vi "HOST_timecycleAIstreaming_11-9.vi"() -> ()   [LabVIEW 2020]
uses:
  <vilib>/rvi/interface/nirviMethod/nirviMethod.xnode
  <vilib>/rvi/errors/niLvFpgaMergeErrorWithErrorCode.vi
  <instrlib>/_niInstr/Streaming/v1/Host/niInstr Streaming v1 Host.lvlib
  <vilib>/rvi/interface/nirviReadWriteControl/nirviReadWriteControl.xnode
  <vilib>/rvi/interface/nirviCloseFPGA/nirviCloseFPGA.xnode
  <vilib>/rvi/interface/nirviOpenFPGA/nirviOpenFPGA.xnode
  <vilib>/rvi/interface/Simulation/niFpgaSimulationCallBeginRW.vi
  <vilib>/rvi/errors/niLvFpgaAdjustHostInterfaceError.vi
  <instrlib>/_niInstr/Streaming/v1/Host/Public/Start Continuous Stream.vi
  <instrlib>/_niInstr/Streaming/v1/Host/Public/Wait for Stream.vi
  <instrlib>/_niInstr/Streaming/v1/Host/Public/Start Finite Stream.vi
  <vilib>/rvi/Analysis/host/Butterworth/config/Butterworth Filter Order.ctl
  <vilib>/rvi/Analysis/host/Public/NI_FpgaMspHost.lvlib
  <vilib>/rvi/Analysis/host/Butterworth/config/Butterworth Filter Type.ctl
  <vilib>/rvi/Analysis/host/Butterworth/config/BwScaledCoefficients.vi
  <vilib>/rvi/Analysis/host/Butterworth/XNode/ButterworthCoefficients.xnode
  FPGA Bitfiles/rfsignal_FPGATarget_TimecyclingNoMod_q9dttbL5ptg.lvbitx
  <vilib>/FPGAPlugInAG/PXIe-7972R/niLvFpga_Open_PXIe-7972R.vi
  <vilib>/rvi/interface/common/dynamic/niFpgaDynamicAddResources.vi
  <vilib>/FPGAPlugInAG/Dynamic/niLvFpga_ConfigureFifo_Dynamic.vi
  <vilib>/FPGAPlugInAG/Dynamic/niLvFpga_StartFifo_Dynamic.vi
  <vilib>/FPGAPlugInAG/Dynamic/niLvFpga_WriteFifo_Dynamic.vi
  <vilib>/FPGAPlugInAG/Dynamic/niLvFpga_ReadFifo_Dynamic.vi
  <vilib>/FPGAPlugInAG/Dynamic/niLvFpga_Close_Dynamic.vi
  <vilib>/userDefined/Silver/nirio_resource_slv.ctl
  Controls/Clock Select.ctl
panel:
  in  "Data Trigger Level (V)":dbl
  in  "Record Size":u16=1024
  out "AI":waveform(dbl)[](graph)
  in  "Data Trigger When":enum8{"Trigger Above", "Trigger Below"}(ring)
  in  "Trigger Type":enum8{"Immediate", "Data Trigger", "TRIG input"}(ring)
  in  "CH0 Amp inc/dec":u8[](array[ring])=[0, 0, 0, 0, 0, 0, 0, 0, 0, 0] items=["", "Increase", "Decrease"]
  in  "CH0 Freq inc/dec":u8[](array[ring])=[0, 0, 0, 0, 0, 0, 0, 0, 0, 0] items=["", "Increase", "Decrease"]
  in  "CH1 Amp inc/dec":u8[](array[ring])=[0, 0, 0, 0, 0, 0, 0, 0, 0, 0] items=["", "Increase", "Decrease"]
  in  "CH1 Freq inc/dec":u8[](array[ring])=[0, 0, 0, 0, 0, 0, 0, 0, 0, 0] items=["", "Increase", "Decrease"]
  in  "LP FF":dbl=5000.0 format="%#_13g"
  in  "Refresh Integral":bool
  in  "Setpoint Z 4":i16
  in  "Lower lim Z 4":fxp<+/-,16,16>=-300.0
  in  "Upper lim Z 4":fxp<+/-,16,16>=300.0
  in  "hp freq Z 4":dbl=1300.0
  in  "lp freq Z 4":dbl=1300.0
  in  "Setpoint Y 4":i16
  in  "Lower lim Y 4":fxp<+/-,16,16>=-300.0
  in  "Upper lim Y 4":fxp<+/-,16,16>=300.0
  in  "hp freq Y 4":dbl=1300.0
  in  "lp freq Y 4":dbl=1300.0
  in  "Setpoint X 4":i16
  in  "Lower lim X 4":fxp<+/-,16,16>=-300.0
  in  "Upper lim X 4":fxp<+/-,16,16>=300.0
  in  "hp freq X 4":dbl=1300.0
  in  "lp freq X 4":dbl=1300.0
  in  "Scaling (Z) 4":fxp<+,16,4>=1.0
  in  "Scaling (Y) 4":fxp<+,16,4>=1.0
  in  "Scaling (X) 4":fxp<+,16,4>=1.0
  in  "D (Z) 4":fxp<+/-,16,16>
  in  "I (Z) 4":fxp<+/-,16,16>
  in  "P (Z) 4":fxp<+/-,16,16>
  in  "D (Y) 4":fxp<+/-,16,16>
  in  "I (Y) 4":fxp<+/-,16,16>
  in  "P (Y) 4":fxp<+/-,16,16>
  in  "D (X) 4":fxp<+/-,16,16>
  in  "I (X) 4":fxp<+/-,16,16>
  in  "P (X) 4":fxp<+/-,16,16>
  in  "Setpoint Z 3":i16
  in  "Lower lim Z 3":fxp<+/-,16,16>=-300.0
  in  "Upper lim Z 3":fxp<+/-,16,16>=300.0
  in  "hp freq Z 3":dbl=1300.0
  in  "lp freq Z 3":dbl=1300.0
  in  "Setpoint Y 3":i16
  in  "Lower lim Y 3":fxp<+/-,16,16>=-300.0
  in  "Upper lim Y 3":fxp<+/-,16,16>=300.0
  in  "hp freq Y 3":dbl=1300.0
  in  "lp freq Y 3":dbl=1300.0
  in  "Setpoint X 3":i16
  in  "Lower lim X 3":fxp<+/-,16,16>=-300.0
  in  "Upper lim X 3":fxp<+/-,16,16>=300.0
  in  "hp freq X 3":dbl=1300.0
  in  "lp freq X 3":dbl=1300.0
  in  "Scaling (Z) 3":fxp<+,16,4>=1.0
  in  "Scaling (Y) 3":fxp<+,16,4>=1.0
  in  "Scaling (X) 3":fxp<+,16,4>=1.0
  in  "D (Z) 3":fxp<+/-,16,16>
  in  "I (Z) 3":fxp<+/-,16,16>
  in  "P (Z) 3":fxp<+/-,16,16>
  in  "D (Y) 3":fxp<+/-,16,16>
  in  "I (Y) 3":fxp<+/-,16,16>
  in  "P (Y) 3":fxp<+/-,16,16>
  in  "D (X) 3":fxp<+/-,16,16>
  in  "I (X) 3":fxp<+/-,16,16>
  in  "P (X) 3":fxp<+/-,16,16>
  in  "Setpoint Z 2":i16
  in  "Lower lim Z 2":fxp<+/-,16,16>=-300.0
  in  "Upper lim Z 2":fxp<+/-,16,16>=300.0
  in  "hp freq Z 2":dbl=1300.0
  in  "lp freq Z 2":dbl=1300.0
  in  "Setpoint Y 2":i16
  in  "Lower lim Y 2":fxp<+/-,16,16>=-300.0
  in  "Upper lim Y 2":fxp<+/-,16,16>=300.0
  in  "hp freq Y 2":dbl=1300.0
  in  "lp freq Y 2":dbl=1300.0
  in  "Setpoint X 2":i16
  in  "Lower lim X 2":fxp<+/-,16,16>=-300.0
  in  "Upper lim X 2":fxp<+/-,16,16>=300.0
  in  "hp freq X 2":dbl=1300.0
  in  "lp freq X 2":dbl=1300.0
  in  "Scaling (Z) 2":fxp<+,16,4>=1.0
  in  "Scaling (Y) 2":fxp<+,16,4>=1.0
  in  "Scaling (X) 2":fxp<+,16,4>=1.0
  in  "D (Z) 2":fxp<+/-,16,16>
  in  "I (Z) 2":fxp<+/-,16,16>
  in  "P (Z) 2":fxp<+/-,16,16>
  in  "D (Y) 2":fxp<+/-,16,16>
  in  "I (Y) 2":fxp<+/-,16,16>
  in  "P (Y) 2":fxp<+/-,16,16>
  in  "D (X) 2":fxp<+/-,16,16>
  in  "I (X) 2":fxp<+/-,16,16>
  in  "P (X) 2":fxp<+/-,16,16>
  in  "Setpoint Z 1":i16
  in  "Lower lim Z 1":fxp<+/-,16,16>=-300.0
  in  "Upper lim Z 1":fxp<+/-,16,16>=300.0
  in  "hp freq Z 1":dbl=1300.0
  in  "lp freq Z 1":dbl=1300.0
  in  "Setpoint Y 1":i16
  in  "Lower lim Y 1":fxp<+/-,16,16>=-300.0
  in  "Upper lim Y 1":fxp<+/-,16,16>=300.0
  in  "hp freq Y 1":dbl=1300.0
  in  "lp freq Y 1":dbl=1300.0
  in  "Setpoint X 1":i16
  in  "Lower lim X 1":fxp<+/-,16,16>=-300.0
  in  "Upper lim X 1":fxp<+/-,16,16>=300.0
  in  "hp freq X 1":dbl=1300.0
  in  "lp freq X 1":dbl=1300.0
  out "AI 2 beam 1":cluster{"AI0":i16, "AI3":i16}(graph)={"AI0"=37, "AI3"=37}
  out "AI 1 beam 1":cluster{"AI0":i16, "AI3":i16}(graph)={"AI0"=-70, "AI3"=-70}
  out "AI 0 beam 1":cluster{"AI0":i16, "AI3":i16}(graph)={"AI0"=-27, "AI3"=-27}
  out "Individual feedback, Z (gain)":cluster{dbl, dbl}(graph)
  out "Individual feedback, Y":cluster{dbl, dbl}(graph)
  out "Individual feedback, X 1":cluster{dbl, dbl}(graph)
  in  "Scaling (Z) 1":fxp<+,16,4>=1.0
  in  "Scaling (Y) 1":fxp<+,16,4>=1.0
  in  "Scaling (X) 1":fxp<+,16,4>=1.0
  in  "D (Z) 1":fxp<+/-,16,16>
  in  "I (Z) 1":fxp<+/-,16,16>
  in  "P (Z) 1":fxp<+/-,16,16>
  in  "D (Y) 1":fxp<+/-,16,16>
  in  "I (Y) 1":fxp<+/-,16,16>
  in  "P (Y) 1":fxp<+/-,16,16>
  in  "D (X) 1":fxp<+/-,16,16>
  in  "I (X) 1":fxp<+/-,16,16>
  in  "P (X) 1":fxp<+/-,16,16>
  out "AI 2 beam 4":cluster{"AI0":i16, "AI3":i16}(graph)
  out "AI 1 beam 4":cluster{"AI0":i16, "AI3":i16}(graph)
  out "AI 0 beam 4":cluster{"AI0":i16, "AI3":i16}(graph)
  out "AI 2 beam 3":cluster{"AI0":i16, "AI3":i16}(graph)={"AI0"=30, "AI3"=30}
  out "AI 1 beam 3":cluster{"AI0":i16, "AI3":i16}(graph)={"AI0"=-64, "AI3"=-64}
  out "AI 0 beam 3":cluster{"AI0":i16, "AI3":i16}(graph)={"AI0"=-28, "AI3"=-28}
  out "AI 2 beam 2":cluster{"AI0":i16, "AI3":i16}(graph)={"AI0"=32, "AI3"=32}
  out "AI 1 beam 2":cluster{"AI0":i16, "AI3":i16}(graph)={"AI0"=-67, "AI3"=-67}
  out "AI 0 beam 2":cluster{"AI0":i16, "AI3":i16}(graph)={"AI0"=-30, "AI3"=-30}
  out "Individual feedback, Z (gain) 4":cluster{dbl, dbl}(graph)
  out "Individual feedback, Z (gain) 3":cluster{dbl, dbl}(graph)
  out "Individual feedback, Z (gain) 2":cluster{dbl, dbl}(graph)
  out "Individual feedback, Y 4":cluster{dbl, dbl}(graph)
  out "Individual feedback, Y 3":cluster{dbl, dbl}(graph)
  out "Individual feedback, Y 2":cluster{dbl, dbl}(graph)
  out "Individual feedback, X 4":cluster{dbl, dbl}(graph)
  out "Individual feedback, X 3":cluster{dbl, dbl}(graph)
  out "Individual feedback, X 2":cluster{dbl, dbl}(graph)
  in  "Norm % 2":dbl=1.0 format="%#_13g"
  in  "Norm %":dbl=1.0 format="%#_13g"
  in  "Amp mod on/off":bool[](array[boolean])=[FALSE, FALSE, FALSE, FALSE, FALSE, FALSE, FALSE, FALSE, FALSE]
  in  "Mod Amp (%)":fxp<+,16,1>[](array[numeric])=[0.5, 1.0, 1.0, 1.0, 0.5, 1.0, 1.0, 1.0, 1.0]
  in  "Mod Fq (Hz) 3":dbl[](array[numeric])=[0.1, 1.0, 1.0, 1.0, 0.1, 1.0, 0.0, 1.0, 1.0] format="%5p"
  in  "Gain X %/s":fxp<+/-,64,32>
  in  "Gain Y %/s":fxp<+/-,64,32>
  in  "X (CH1) Hz/s":fxp<+/-,64,32>
  in  "Y (CH0) Hz/s":fxp<+/-,64,32>
  in  "Input pass through\nmode":enum16{"Wire", "Accum", "Accum-edge"}(ring)
  in  "# of beams":i8=1
  in  "Wave Reader CH 1 (X)":fxp<+/-,64,32>[](array[numeric])=[27000000.0, 26000000.0, 28000000.0, 25000000.0, 21000000.0, 25000000.0, 30000000.0, 34000000.0, 27000000.0] format="%_17p"
  in  "Gain CH 1 (multiplicative)":fxp<+,32,4>[](array[numeric])=[1.0, 1.0, 0.9999999925494194, 1.0, 1.0, 1.0, 1.0, 1.0, 1.0]
  in  "Remove transition edges":i32=5
  in  "Time per beam in us":i32=20
  in  "stop":bool
  in  "Gain CH 0 (multiplicative)":fxp<+,32,4>[](array[numeric])=[1.0, 1.0, 1.0, 1.0, 1.0, 1.0, 1.0, 1.0, 1.0]
  in  "Wave Reader CH 0 (Y)":fxp<+/-,64,32>[](array[numeric])=[27000000.0, 26000000.0, 28000000.0, 25000000.0, 21000000.0, 25000000.0, 30000000.0, 34000000.0, 27000000.0] format="%_17p"
  out "AO":waveform(dbl)(graph)={"t0"=timestamp(0.0004 s since 1904-01-01), "dt"=6.103515625e-09, "Y"=array[65536 elements]}
  in  "Magnitude Initialization Vpp":dbl[](array[numeric])=[1.0, 1.0] format="%0.2p"
  in  "Frequencies (Hz)":dbl[](array[numeric])=[10000.0, 10000.0] format="%5.0p"
  in  "Signal Type":T1(ring)
  in  "Sampling Info":cluster{"Fs":dbl, "#s":dbl}={"Fs"=163840000.0, "#s"=65536.0} {"Fs" format="%#_5p"}
  out "Error Out":errorcluster
  in  "Update Waveform":bool
  in  "AO Channel":T2(ring)
  in  "Clock Select":T3 items=["Internal Clock", "Internal Clock w/ Ref via CLK/REF IN", "Internal Clock w/ Ref via Sync Clock", "External Clock via CLK/REF IN"]
  in  "Rate of External Sample Clock (MHz)":u16=100 min=60 max=100 step=1
  in  "RIO Resource":T4="PXI1Slot5"
  # "AI Configuration"
  # "Don't change"
  # "Waveform Initialization"
  # "DO NOT CHANGE"
  # "Ch 0 Output Waveforms"
  # "Ch 1 Output Waveforms"
  # "Amplitude Sin Modulation"
  # "General Feedback Settings"
  # "Time cycle loop processing"
  # "Shared Feedback Controls"
  # "Initialization waveform stored in FPGA"
  # "Ch0"
  # "Ch1"
  # "Beam 1 Feedback Parameters"
  # "Beam 2 Feedback Parameters"
  # "Beam 3 Feedback Parameters"
  # "Beam 4 Feedback Parameters"
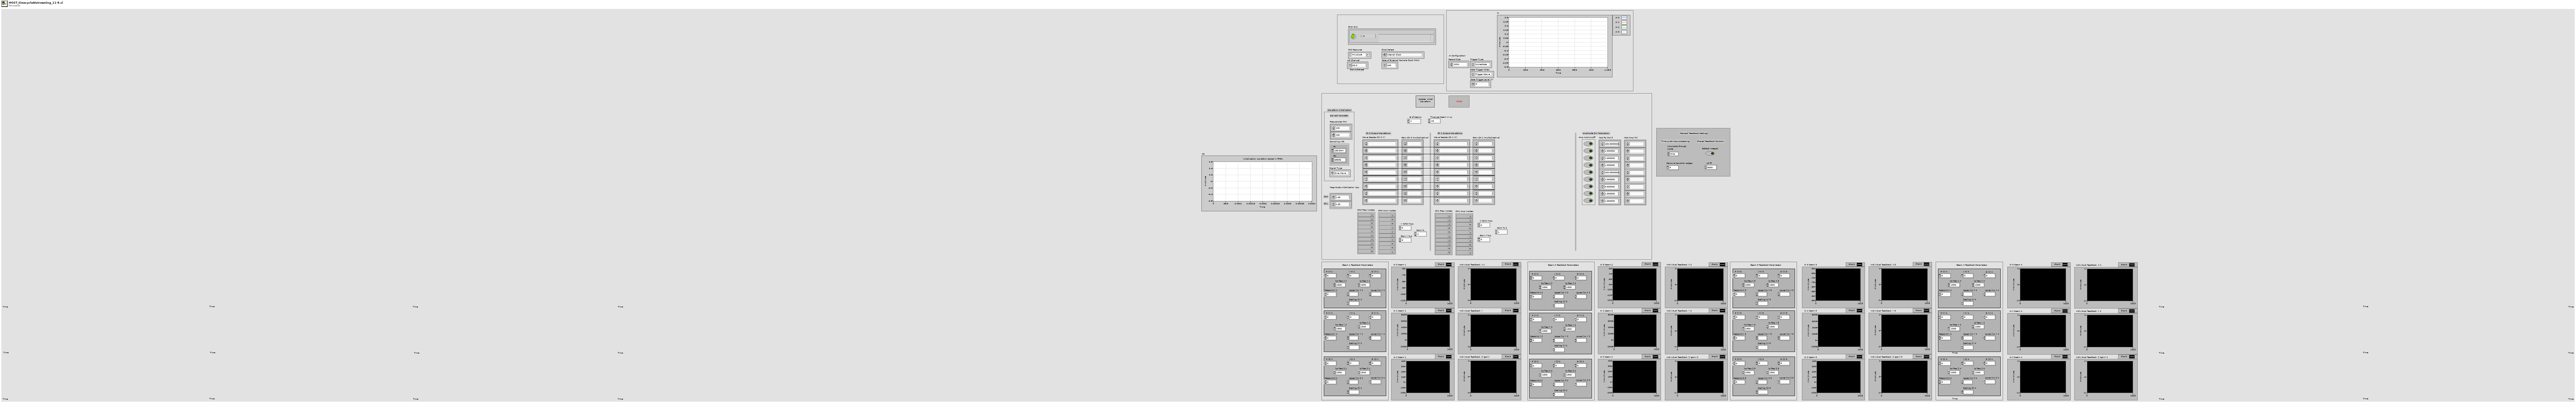
[diagram p1: front panel]
types:
  T1 = enum16{"Sine Wave", "Triangle Wave", "Square Wave", "Sawtooth Wave"}
  T2 = enum8{"AO 0", "AO 1", "AO 2", "AO 3", "AO 0, AO 1, AO 2, AO 3", "None"}
  T3 = typedef "Clock Select.ctl" = u16
  T4 = typedef "nirio_resource_slv.ctl" = tag
  T5 = cluster{"AI 0 input 1":void, "AI 0 input 1":void}
  T6 = cluster{"AI 1 input 1":void, "AI 1 input 1":void}
  T7 = cluster{"AI 2 input 1":void, "AI 2 input 1":void}
  T8 = cluster{"AI 0 input 2":void, "AI 0 input 2":void}
  T9 = cluster{"AI 1 input 2":void, "AI 1 input 2":void}
  T10 = cluster{"AI 2 input 2":void, "AI 2 input 2":void}
  T11 = cluster{"AI 0 input 3":void, "AI 0 input 3":void}
  T12 = cluster{"AI 1 input 3":void, "AI 1 input 3":void}
  T13 = cluster{"AI 0 input 4":void, "AI 0 input 4":void}
  T14 = cluster{"AI 2 input 3":void, "AI 2 input 3":void}
  T15 = cluster{"AI 1 input 4":void, "AI 1 input 4":void}
  T16 = cluster{"AI 2 input 4":void, "AI 2 input 4":void}
  T17 = cluster{"level":i16, "trigger when":enum8{"Trigger Above", "Trigger Below"}}
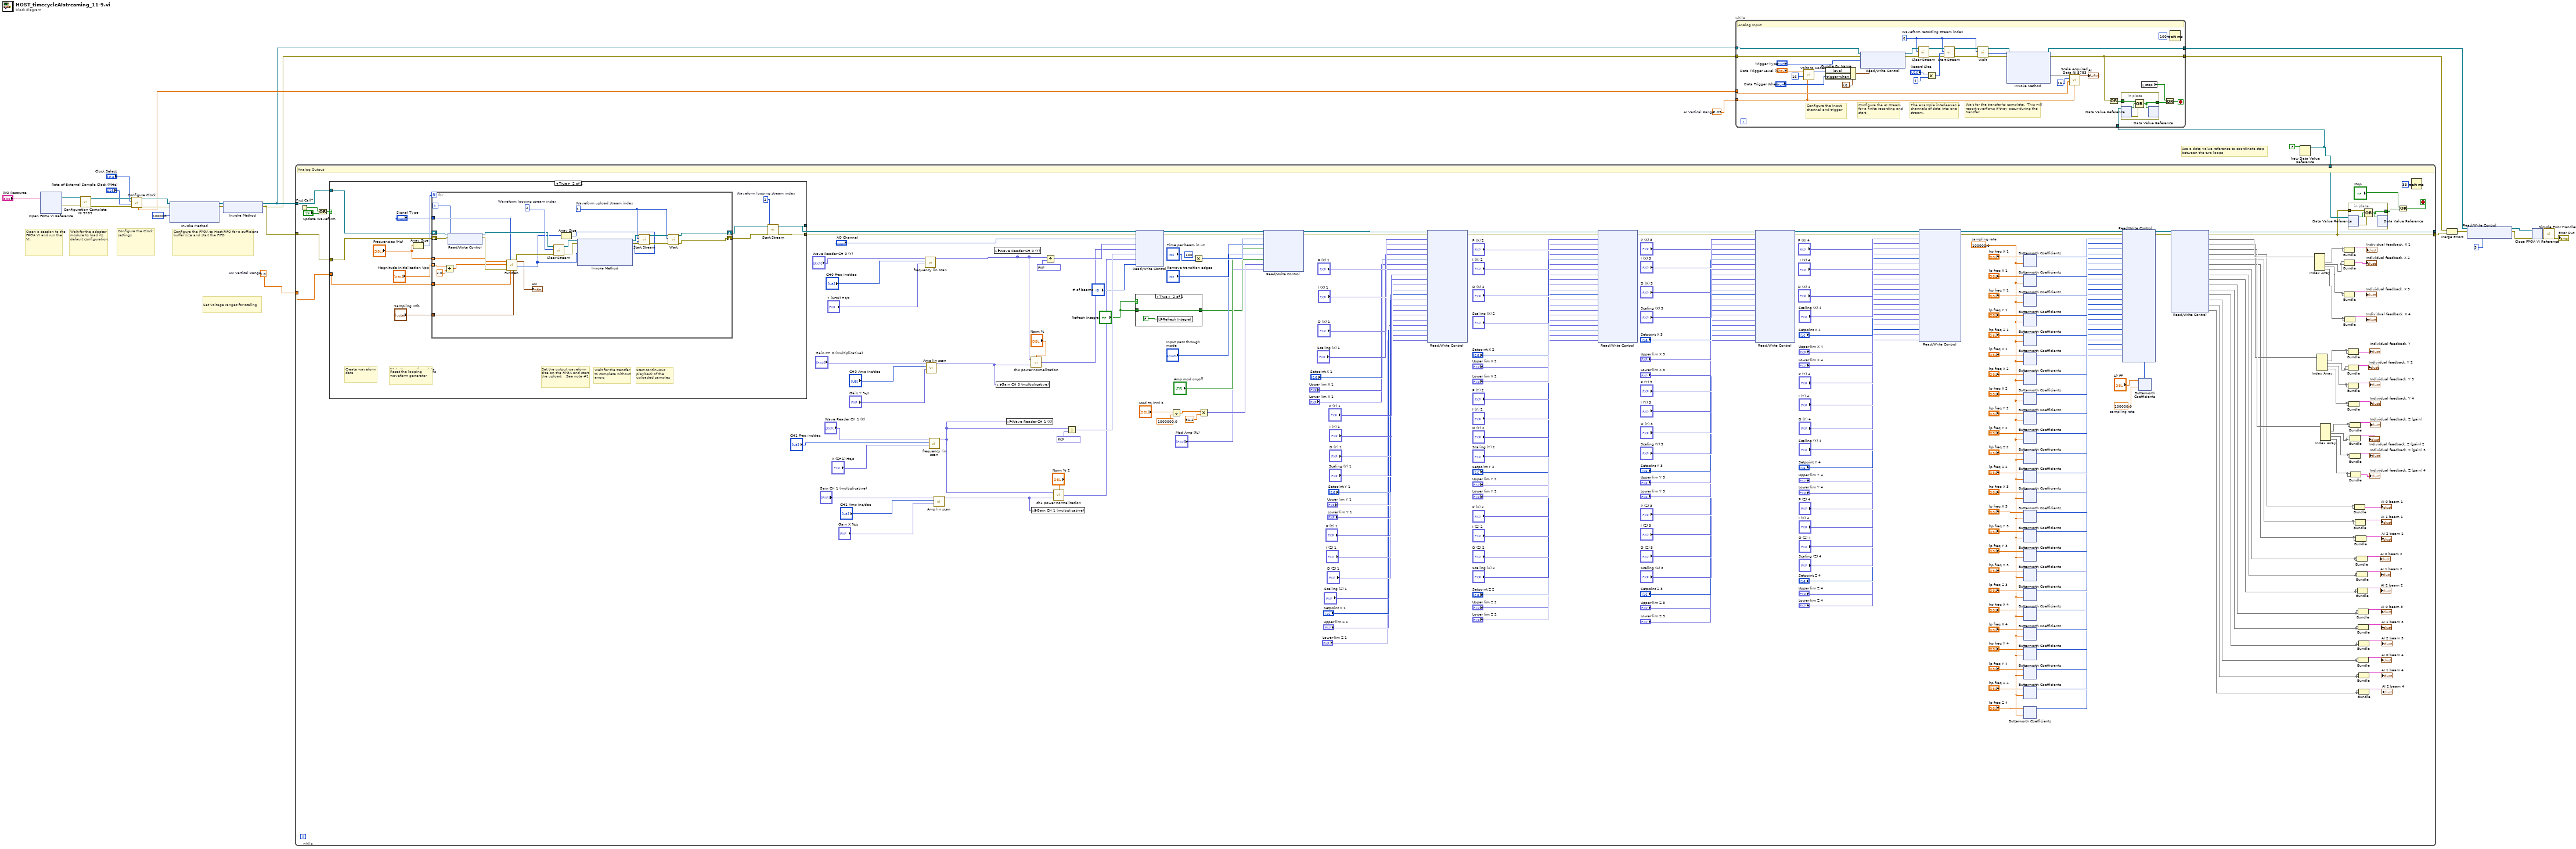
[diagram p0: block diagram]
diagram:
  w8 = 2.03  # AI Vertical Range
  w16 = 1.0  # AO Vertical Range
  # "Use a data value reference to coordinate stop between the two loops"
  # "Set Voltage ranges for scaling"
  # "Configure the Clock settings"
  # "Configure the FPGA to Host FIFO for a sufficient buffer size and start the FIFO"
  # "Wait for the adapter module to load its default configuration."
  # "Open a session to the FPGA VI and run the VI."
  n1 = xnode "Open FPGA VI Reference"("resource name"="RIO Resource") -> ("FPGA VI Reference Out"=w14:refnum<k20>, "error out"=w13:errorcluster)  [unwired: 1 in]
  n2 = call "Configuration Complete NI 5783.vi"("error in"=w13, "FPGA VI Reference In"=w14) -> ("error out"=w24:errorcluster, "FPGA VI Reference Out"=w25:refnum<k20>)  [unwired: 7 in, 1 out]
  n3 = call "Configure Clock.vi"("error in (no error)"=w24, "Rate of External Sample Clock (MHz)"="Rate of External Sample Clock (MHz)", "Clock Select"="Clock Select", "FPGA VI Reference In"=w25) -> ("error out"=w22:errorcluster, "FPGA VI Reference Out"=w23:refnum<k20>, "Sampling Rate"=w7:dbl)  [unwired: 3 in, 2 out]
  n4 = xnode "Invoke Method"("FPGA VI Reference In"=w23, "error in"=w22, "Requested Depth"=u32 100000) -> ("FPGA VI Reference Out"=w28:refnum<k20>, "error out"=w27:errorcluster)  [unwired: 1 out]
  n5 = xnode "Invoke Method"("FPGA VI Reference In"=w28, "error in"=w27) -> ("FPGA VI Reference Out"=w6:refnum<k20>, "error out"=w5:errorcluster)
  n6 = New Data Value Reference(data value=FALSE ("Stopped")) -> (data value reference=w9:refnum<data-value>)  [unwired: 1 in, 1 out]
  n7 = while {
    tunnel: w5 -> [w278]
    tunnel: [w239] -> w2
    tunnel: w6 -> [w284]
    tunnel: [w72] -> _
    tunnel: w9 -> [w279]
    tunnel: w16 -> [w277]
    stop <- w273 stop-if-true
    w41 = 100000.0  # sampling rate
    w73 = 100000.0  # sampling rate
    # "Analog Output"
    n8 = First Call?() -> (First Call?: T/F=w280:bool)
    n9 = Or(x=w280, y="Update Waveform") -> (x .or. y?=w281:bool)
    n10 = case shown="True" w281 {
      tunnel: [w468 w481] -> w276
      tunnel: [w467 w480] -> w275
      tunnel: w284 -> [w468 w478]
      tunnel: w278 -> [w467 w477]
      tunnel: w277 -> [_ w479]
      frame False {
      }
      frame True {
        w476 = 2  # Waveform looping stream index
        # "Loop over the waveforms to combine"
        # "Reset the looping waveform generator"
        # "Start continuous playback of the uploaded samples"
        # "Wait for the transfer to complete without errors"
        # "Set the output waveform size on the FPGA and start the upload.   See note #1"
        # "Write the waveform data to the FPGA for generation"
        # "Create waveform data"
        n11 = Array Size(array="Frequencies (Hz)") -> (size(s)=w471:i32)
        n12 = for {
          N: w471 -> [_]
          tunnel: w479 -> [w497]
          shift-right: [w491] -> w475
          shift-left: w478 -> [w496]
          shift-right: [w490] -> w474
          shift-left: w477 -> [w494]
          tunnel: "Frequencies (Hz)" -> [w489] mode=indexing
          tunnel: "Magnitude Initialization Vpp" -> [w485] mode=indexing
          tunnel: "Sampling Info" -> [w488]
          tunnel: "Signal Type" -> [w487]
          i -> [w486]
          w498 = 2  # Waveform looping stream index
          w503 = 1  # Waveform upload stream index
          n13 = Divide(x=w485, y=2.0) -> (x/y=w484:dbl)
          n14 = xnode "Read/Write Control"("FPGA VI Reference In"=w496, "error in"=w494, "Upload selector"=w486) -> ("FPGA VI Reference Out"=w495:refnum<k20>, "error out"=w493:errorcluster)
          n15 = call "FunGen.vi"("sampling info"=w488, "range (Vpp)"=w497, "signal type"=w487, "error in (no error)"=w493, "amplitude"=w484, "frequency"=w489) -> ("error out"=w499:errorcluster, "Waveform Data"=w492:i16[], "Output Waveform (V)"=→"AO":waveform(dbl))  [unwired: 2 in, 1 out]
          n16 = call <instrlib>:"Clear Stream.vi"("error in (no error)"=w499, "stream index"=w498, "refnum in"=w495) -> ("error out"=w501:errorcluster, "refnum out"=w502:refnum<k20>)  [unwired: 7 in]
          n17 = Array Size(array=w492) -> (size(s)=w500:i32)
          n18 = xnode "Invoke Method"("FPGA VI Reference In"=w502, "error in"=w501, "Data"=w492) -> ("FPGA VI Reference Out"=w507:refnum<k20>, "error out"=w506:errorcluster)  [unwired: 1 in, 1 out]
          n19 = call-poly <instrlib>:"Start Stream.vi"("error in (no error)"=w506, "num samples"=w500, "stream index"=w503, "refnum in"=w507) -> ("error out"=w504:errorcluster, "refnum out"=w505:refnum<k20>)  [unwired: 6 in]
          n20 = call-poly <instrlib>:"Wait.vi"("error in (no error)"=w504, "stream index"=w503, "refnum in"=w505) -> ("error out"=w490:errorcluster, "refnum out"=w491:refnum<k20>)  [unwired: 5 in, 2 out]
        }
        n21 = call-poly <instrlib>:"Start Stream.vi"("error in (no error)"=w474, "stream index"=w476, "refnum in"=w475) -> ("error out"=w480:errorcluster, "refnum out"=w481:refnum<k20>)  [unwired: 7 in]
      }
    }
    n22 = call "frequency lin scan.vi"("Hz/s"="Y (CH0) Hz/s", "Freq inc/dec"="CH0 Freq inc/dec", "Wave Reader"="Wave Reader CH 0 (Y)") -> ("Array"=w37:fxp<+/-,64,32>[])  [unwired: 8 in]
    n23 = call "Amp lin scan.vi"("Gain %/s"="Gain Y %/s", "Amp inc/dec"="CH0 Amp inc/dec", "Gain"="Gain CH 0 (multiplicative)") -> ("Array"=w32:fxp<+,32,4>[])  [unwired: 8 in]
    n24 = call "frequency lin scan.vi"("Hz/s"="X (CH1) Hz/s", "Freq inc/dec"="CH1 Freq inc/dec", "Wave Reader"="Wave Reader CH 1 (X)") -> ("Array"=w243:fxp<+/-,64,32>[])  [unwired: 8 in]
    n25 = call "Amp lin scan.vi"("Gain %/s"="Gain X %/s", "Amp inc/dec"="CH1 Amp inc/dec", "Gain"="Gain CH 1 (multiplicative)") -> ("Array"=w245:fxp<+,32,4>[])  [unwired: 8 in]
    n26 = local write "Wave Reader CH 0 (Y)"(w37) -> ()
    n27 = local write "Gain CH 0 (multiplicative)"(w32) -> ()
    n28 = local write "Wave Reader CH 1 (X)"(w243) -> ()
    n29 = call "ch0 power normalization.vi"("% of max"="Norm %", "Gain"=w32, "Wave freq"=w37) -> ("Array"=w241:fxp<+,32,2>[])
    n30 = local write "Gain CH 1 (multiplicative)"(w245) -> ()
    n31 = Divide(x=w37, y=fxp<+,32,16> 6103.515625) -> (x/y=w264:fxp<+,34,16>[])
    n32 = call "ch1 power normalization.vi"("% of max"="Norm % 2", "Gain"=w245, "Wave freq"=w243) -> ("Array"=w244:fxp<+,32,2>[])
    n33 = Divide(x=w243, y=fxp<+,32,16> 6103.515625) -> (x/y=w262:fxp<+,34,16>[])
    n34 = case shown="True" "Refresh Integral" {
      tunnel: [w285 w286] -> w40
      tunnel: "Refresh Integral" -> [w285 w286]
      frame False {
      }
      frame True {
        n35 = local write "Refresh Integral"(FALSE) -> ()
      }
    }
    n36 = xnode "Read/Write Control"("FPGA VI Reference In"=w276, "error in"=w275, "AO Channel"="AO Channel", "Wave 1"=w264, "Amp Set 1"=w241, "Wave 2"=w262, "Amp 2"=w244, "Size"="# of beams") -> ("FPGA VI Reference Out"=w269:refnum<k20>, "error out"=w268:errorcluster)
    n37 = Divide(x="Mod Fq (Hz) 3", y=1000000.0) -> (x/y=w250:dbl[])
    n38 = Multiply(x=100, y="Time per beam in us") -> (x*y=w265:i32)
    n39 = Multiply(x=w250, y=51.2) -> (x*y=w247:fxp<+,32,13>[])
    n40 = xnode "Read/Write Control"("FPGA VI Reference In"=w269, "error in"=w268, "Timeshare"=w265, "Edge size"="Remove transition edges", "Integral reset"=w40, "Pass selector"="Input pass through\nmode", "Amp mod (on/off)"="Amp mod on/off", "Amp mod f"=w247, "Amp mod gain"="Mod Amp (%)") -> ("FPGA VI Reference Out"=w254:refnum<k20>, "error out"=w253:errorcluster)
    n41 = xnode "Read/Write Control"("FPGA VI Reference In"=w254, "error in"=w253, "Px gain 1"="P (X) 1", "Ix gain 1"="I (X) 1", "Dx gain 1"="D (X) 1", "Feedback scaling 2"="Scaling (X) 1", "X DC offset 1"="Setpoint X 1", "X up lim 1"="Upper lim X 1", "X low lim 1"="Lower lim X 1", "Py gain 1"="P (Y) 1", "Iy gain 1"="I (Y) 1", "Dy gain 1"="D (Y) 1", "Feedback scaling"="Scaling (Y) 1", "Y DC offset 1"="Setpoint Y 1", "Y up lim 1"="Upper lim Y 1", "Y low lim 1"="Lower lim Y 1", "P_amp gain 1"="P (Z) 1", "I_amp gain 1"="I (Z) 1", "D_amp gain 1"="D (Z) 1", "Feedback scaling 3"="Scaling (Z) 1", "Z DC offset 1"="Setpoint Z 1", "Amp up lim 1"="Upper lim Z 1", "Amp low lim 1"="Lower lim Z 1") -> ("FPGA VI Reference Out"=w181:refnum<k20>, "error out"=w180:errorcluster)
    n42 = xnode "Read/Write Control"("FPGA VI Reference In"=w181, "error in"=w180, "Px gain 2"="P (X) 2", "Ix gain 2"="I (X) 2", "Dx gain 2"="D (X) 2", "Feedback scaling 5"="Scaling (X) 2", "X DC offset 2"="Setpoint X 2", "X up lim 2"="Upper lim X 2", "X low lim 2"="Lower lim X 2", "Py gain 2"="P (Y) 2", "Iy gain 2"="I (Y) 2", "Dy gain 2"="D (Y) 2", "Feedback scaling 4"="Scaling (Y) 2", "Y DC offset 2"="Setpoint Y 2", "Y up lim 2"="Upper lim Y 2", "Y low lim 2"="Lower lim Y 2", "P_amp gain 2"="P (Z) 2", "I_amp gain 2"="I (Z) 2", "D_amp gain 3"="D (Z) 2", "Feedback scaling 6"="Scaling (Z) 2", "Z DC offset 2"="Setpoint Z 2", "Amp up lim 2"="Upper lim Z 2", "Amp low lim 2"="Lower lim Z 2") -> ("FPGA VI Reference Out"=w158:refnum<k20>, "error out"=w156:errorcluster)
    n43 = xnode "Read/Write Control"("FPGA VI Reference In"=w158, "error in"=w156, "Px gain 3"="P (X) 3", "Ix gain 3"="I (X) 3", "Dx gain 3"="D (X) 3", "Feedback scaling 8"="Scaling (X) 3", "X DC offset 3"="Setpoint X 3", "X up lim 3"="Upper lim X 3", "X low lim 3"="Lower lim X 3", "Py gain 3"="P (Y) 3", "Iy gain 3"="I (Y) 3", "Dy gain 3"="D (Y) 3", "Feedback scaling 7"="Scaling (Y) 3", "Y DC offset 3"="Setpoint Y 3", "Y up lim 3"="Upper lim Y 3", "Y low lim 3"="Lower lim Y 3", "P_amp gain 3"="P (Z) 3", "I_amp gain 3"="I (Z) 3", "D_amp gain 3"="D (Z) 3", "Feedback scaling 9"="Scaling (Z) 3", "Z DC offset 3"="Setpoint Z 3", "Amp up lim 3"="Upper lim Z 3", "Amp low lim 3"="Lower lim Z 3") -> ("FPGA VI Reference Out"=w89:refnum<k20>, "error out"=w157:errorcluster)
    n44 = xnode "Read/Write Control"("FPGA VI Reference In"=w89, "error in"=w157, "Px gain 4"="P (X) 4", "Ix gain 4"="I (X) 4", "Dx gain 4"="D (X) 4", "Feedback scaling 11"="Scaling (X) 4", "X DC offset 4"="Setpoint X 4", "X up lim 4"="Upper lim X 4", "X low lim 4"="Lower lim X 4", "Py gain 4"="P (Y) 4", "Iy gain 4"="I (Y) 4", "Dy gain 4"="D (Y) 4", "Feedback scaling 10"="Scaling (Y) 4", "Y DC offset 4"="Setpoint Y 4", "Y up lim 4"="Upper lim Y 4", "Y low lim 4"="Lower lim Y 4", "P_amp gain 4"="P (Z) 4", "I_amp gain 4"="I (Z) 4", "D_amp gain 4"="D (Z) 4", "Feedback scaling 12"="Scaling (Z) 4", "Z DC offset 4"="Setpoint Z 4", "Amp up lim 4"="Upper lim Z 4", "Amp low lim 4"="Lower lim Z 4") -> ("FPGA VI Reference Out"=w71:refnum<k20>, "error out"=w69:errorcluster)
    n45 = xnode "Butterworth Coefficients"("cutoff frequency (Hz)"="hp freq X 1", "sample rate (S/s)"=w73) -> ("scaled coefficients"=w68:i32[])  [unwired: 1 in, 1 out]
    n46 = xnode "Butterworth Coefficients"("cutoff frequency (Hz)"="lp freq X 1", "sample rate (S/s)"=w73) -> ("scaled coefficients"=w67:i32[])  [unwired: 1 in, 1 out]
    n47 = xnode "Butterworth Coefficients"("cutoff frequency (Hz)"="hp freq Y 1", "sample rate (S/s)"=w73) -> ("scaled coefficients"=w66:i32[])  [unwired: 1 in, 1 out]
    n48 = xnode "Butterworth Coefficients"("cutoff frequency (Hz)"="lp freq Y 1", "sample rate (S/s)"=w73) -> ("scaled coefficients"=w65:i32[])  [unwired: 1 in, 1 out]
    n49 = xnode "Butterworth Coefficients"("cutoff frequency (Hz)"="hp freq Z 1", "sample rate (S/s)"=w73) -> ("scaled coefficients"=w64:i32[])  [unwired: 1 in, 1 out]
    n50 = xnode "Butterworth Coefficients"("cutoff frequency (Hz)"="lp freq Z 1", "sample rate (S/s)"=w73) -> ("scaled coefficients"=w63:i32[])  [unwired: 1 in, 1 out]
    n51 = xnode "Butterworth Coefficients"("cutoff frequency (Hz)"="hp freq X 2", "sample rate (S/s)"=w73) -> ("scaled coefficients"=w62:i32[])  [unwired: 1 in, 1 out]
    n52 = xnode "Butterworth Coefficients"("cutoff frequency (Hz)"="lp freq X 2", "sample rate (S/s)"=w73) -> ("scaled coefficients"=w61:i32[])  [unwired: 1 in, 1 out]
    n53 = xnode "Butterworth Coefficients"("cutoff frequency (Hz)"="hp freq Y 2", "sample rate (S/s)"=w73) -> ("scaled coefficients"=w60:i32[])  [unwired: 1 in, 1 out]
    n54 = xnode "Butterworth Coefficients"("cutoff frequency (Hz)"="lp freq Y 2", "sample rate (S/s)"=w73) -> ("scaled coefficients"=w59:i32[])  [unwired: 1 in, 1 out]
    n55 = xnode "Butterworth Coefficients"("cutoff frequency (Hz)"="hp freq Z 2", "sample rate (S/s)"=w73) -> ("scaled coefficients"=w58:i32[])  [unwired: 1 in, 1 out]
    n56 = xnode "Butterworth Coefficients"("cutoff frequency (Hz)"="lp freq Z 2", "sample rate (S/s)"=w73) -> ("scaled coefficients"=w57:i32[])  [unwired: 1 in, 1 out]
    n57 = xnode "Butterworth Coefficients"("cutoff frequency (Hz)"="hp freq X 3", "sample rate (S/s)"=w73) -> ("scaled coefficients"=w56:i32[])  [unwired: 1 in, 1 out]
    n58 = xnode "Butterworth Coefficients"("cutoff frequency (Hz)"="lp freq X 3", "sample rate (S/s)"=w73) -> ("scaled coefficients"=w55:i32[])  [unwired: 1 in, 1 out]
    n59 = xnode "Butterworth Coefficients"("cutoff frequency (Hz)"="hp freq Y 3", "sample rate (S/s)"=w73) -> ("scaled coefficients"=w54:i32[])  [unwired: 1 in, 1 out]
    n60 = xnode "Butterworth Coefficients"("cutoff frequency (Hz)"="lp freq Y 3", "sample rate (S/s)"=w73) -> ("scaled coefficients"=w53:i32[])  [unwired: 1 in, 1 out]
    n61 = xnode "Butterworth Coefficients"("cutoff frequency (Hz)"="hp freq Z 3", "sample rate (S/s)"=w73) -> ("scaled coefficients"=w52:i32[])  [unwired: 1 in, 1 out]
    n62 = xnode "Butterworth Coefficients"("cutoff frequency (Hz)"="lp freq Z 3", "sample rate (S/s)"=w73) -> ("scaled coefficients"=w51:i32[])  [unwired: 1 in, 1 out]
    n63 = xnode "Butterworth Coefficients"("cutoff frequency (Hz)"="hp freq X 4", "sample rate (S/s)"=w73) -> ("scaled coefficients"=w50:i32[])  [unwired: 1 in, 1 out]
    n64 = xnode "Butterworth Coefficients"("cutoff frequency (Hz)"="lp freq X 4", "sample rate (S/s)"=w73) -> ("scaled coefficients"=w48:i32[])  [unwired: 1 in, 1 out]
    n65 = xnode "Butterworth Coefficients"("cutoff frequency (Hz)"="hp freq Y 4", "sample rate (S/s)"=w73) -> ("scaled coefficients"=w47:i32[])  [unwired: 1 in, 1 out]
    n66 = xnode "Butterworth Coefficients"("cutoff frequency (Hz)"="lp freq Y 4", "sample rate (S/s)"=w73) -> ("scaled coefficients"=w46:i32[])  [unwired: 1 in, 1 out]
    n67 = xnode "Butterworth Coefficients"("cutoff frequency (Hz)"="hp freq Z 4", "sample rate (S/s)"=w73) -> ("scaled coefficients"=w45:i32[])  [unwired: 1 in, 1 out]
    n68 = xnode "Butterworth Coefficients"("cutoff frequency (Hz)"="lp freq Z 4", "sample rate (S/s)"=w73) -> ("scaled coefficients"=w44:i32[])  [unwired: 1 in, 1 out]
    n69 = xnode "Butterworth Coefficients"("cutoff frequency (Hz)"="LP FF", "sample rate (S/s)"=w41) -> ("scaled coefficients"=w43:i32[])  [unwired: 1 in, 1 out]
    n70 = xnode "Read/Write Control"("FPGA VI Reference In"=w71, "error in"=w69, "X hp coef 1"=w68, "X lp coef 1"=w67, "Y hp coef 1"=w66, "Y lp coef 1"=w65, "Z hp coef 1"=w64, "Z lp coef 1"=w63, "X hp coef 2"=w62, "X lp coef 2"=w61, "Y hp coef 2"=w60, "Y lp coef 2"=w59, "Z hp coef 2"=w58, "Z lp coef 2"=w57, "X hp coef 3"=w56, "X lp coef 3"=w55, "Y hp coef 3"=w54, "Y lp coef 3"=w53, "Z hp coef 3"=w52, "Z lp coef 3"=w51, "X hp coef 4"=w50, "X lp coef 4"=w48, "Y hp coef 4"=w47, "Y lp coef 4"=w46, "Z hp coef 4"=w45, "Z lp coef 4"=w44, "Final filter coef"=w43) -> ("FPGA VI Reference Out"=w70:refnum<k20>, "error out"=w49:errorcluster)
    n71 = xnode "Read/Write Control"("FPGA VI Reference In"=w70, "error in"=w49) -> ("FPGA VI Reference Out"=w72:refnum<k20>, "error out"=w239:errorcluster, "Feedback x (CH1)"=w88, "Feedback y (CH0)"=w86, "Feedback z (amp)"=w87, "AI 0 input 1"=w85, "AI 1 input 1"=w84, "AI 2 input 1"=w83, "AI 0 input 2"=w82, "AI 1 input 2"=w81, "AI 2 input 2"=w80, "AI 0 input 3"=w79, "AI 1 input 3"=w78, "AI 2 input 3"=w77, "AI 0 input 4"=w76, "AI 1 input 4"=w75, "AI 2 input 4"=w74)
    n72 = Index Array(array=w88) -> (element #1=w238, element #2=w234, element #3=w233, element #4=w232)  [unwired: 4 in]
    n73 = Index Array(array=w86) -> (element #1=w231, element #2=w230, element #3=w229, element #4=w228)  [unwired: 4 in]
    n74 = Index Array(array=w87) -> (element #1=w224, element #2=w223, element #3=w222, element #4=w221)  [unwired: 4 in]
    n75 = Bundle(w238, w238) -> (→"Individual feedback, X 1":cluster{void, void})  [unwired: 1 in]
    n76 = Bundle(w234, w234) -> (→"Individual feedback, X 2":cluster{void, void})  [unwired: 1 in]
    n77 = Bundle(w233, w233) -> (→"Individual feedback, X 3":cluster{void, void})  [unwired: 1 in]
    n78 = Bundle(w232, w232) -> (→"Individual feedback, X 4":cluster{void, void})  [unwired: 1 in]
    n79 = in-place {
      in-place-border: [w464] -> w272
      in-place-border: w239 -> [w466]
      n80 = in-place-dvr #1(w279) -> (w465:bool, w463:errorcluster)
      n81 = Compound Arithmetic op=OR(w466, w465, w463) -> (w464:bool)
      n82 = in-place-dvr #1(w464) -> ()  [unwired: 2 out]
    }
    n83 = Bundle(w231, w231) -> (→"Individual feedback, Y":cluster{void, void})  [unwired: 1 in]
    n84 = Bundle(w230, w230) -> (→"Individual feedback, Y 2":cluster{void, void})  [unwired: 1 in]
    n85 = Bundle(w229, w229) -> (→"Individual feedback, Y 3":cluster{void, void})  [unwired: 1 in]
    n86 = Bundle(w228, w228) -> (→"Individual feedback, Y 4":cluster{void, void})  [unwired: 1 in]
    n87 = Bundle(w224, w224) -> (→"Individual feedback, Z (gain)":cluster{void, void})  [unwired: 1 in]
    n88 = Bundle(w223, w223) -> (→"Individual feedback, Z (gain) 2":cluster{void, void})  [unwired: 1 in]
    n89 = Bundle(w222, w222) -> (→"Individual feedback, Z (gain) 3":cluster{void, void})  [unwired: 1 in]
    n90 = Bundle(w221, w221) -> (→"Individual feedback, Z (gain) 4":cluster{void, void})  [unwired: 1 in]
    n91 = Bundle("AI 0 input 1"=w85, "AI 0 input 1"=w85) -> (→"AI 0 beam 1":T5)  [unwired: 1 in]
    n92 = Bundle("AI 1 input 1"=w84, "AI 1 input 1"=w84) -> (→"AI 1 beam 1":T6)  [unwired: 1 in]
    n93 = Bundle("AI 2 input 1"=w83, "AI 2 input 1"=w83) -> (→"AI 2 beam 1":T7)  [unwired: 1 in]
    n94 = Bundle("AI 0 input 2"=w82, "AI 0 input 2"=w82) -> (→"AI 0 beam 2":T8)  [unwired: 1 in]
    n95 = Bundle("AI 1 input 2"=w81, "AI 1 input 2"=w81) -> (→"AI 1 beam 2":T9)  [unwired: 1 in]
    n96 = Bundle("AI 2 input 2"=w80, "AI 2 input 2"=w80) -> (→"AI 2 beam 2":T10)  [unwired: 1 in]
    n97 = Bundle("AI 0 input 3"=w79, "AI 0 input 3"=w79) -> (→"AI 0 beam 3":T11)  [unwired: 1 in]
    n98 = Bundle("AI 1 input 3"=w78, "AI 1 input 3"=w78) -> (→"AI 1 beam 3":T12)  [unwired: 1 in]
    n99 = Bundle("AI 0 input 4"=w76, "AI 0 input 4"=w76) -> (→"AI 0 beam 4":T13)  [unwired: 1 in]
    n100 = Bundle("AI 2 input 3"=w77, "AI 2 input 3"=w77) -> (→"AI 2 beam 3":T14)  [unwired: 1 in]
    n101 = Bundle("AI 1 input 4"=w75, "AI 1 input 4"=w75) -> (→"AI 1 beam 4":T15)  [unwired: 1 in]
    n102 = Bundle("AI 2 input 4"=w74, "AI 2 input 4"=w74) -> (→"AI 2 beam 4":T16)  [unwired: 1 in]
    n103 = Or(x="stop", y=w272) -> (x .or. y?=w273:bool)
    n104 = Wait (ms)(milliseconds to wait=u32 33) -> ()  [unwired: 1 out]
  }
  n105 = while {
    tunnel: [w541] -> w4
    tunnel: w8 -> [w521]
    tunnel: w9 -> [w539]
    tunnel: w5 -> [w540]
    tunnel: [w527] -> w1
    tunnel: w7 -> [w522]
    tunnel: w6 -> [w508]
    stop <- w511 stop-if-true
    w512 = 0  # Waveform recording stream index
    # "The example interleaves 4 channels of data into one stream."
    # "Wait for the transfer to complete.  This will report overflows if they occur during the transfer."
    # "Configure the AI stream for a finite recording and start"
    # "Configure the input channel and trigger"
    # "Analog Input"
    n106 = call "Volts to Codes.vi"("range (Vpp)"=w521, "Number of Bits"=i16 16, "Volts In"="Data Trigger Level (V)") -> ("ADC Codes Out"=w523:i16)  [unwired: 8 in]
    n107 = Bundle By Name(cluster=T17 {"level"=0, "trigger when"=enum."Trigger Above"} ("Trigger Configuration"), "level"=w523, "trigger when"="Data Trigger When") -> (w526:T17)
    n108 = xnode "Read/Write Control"("FPGA VI Reference In"=w508, "error in"=w540, "Trigger Type"="Trigger Type", "Trigger Configuration"=w526) -> ("FPGA VI Reference Out"=w516:refnum<k20>, "error out"=w515:errorcluster)
    n109 = call <instrlib>:"Clear Stream.vi"("error in (no error)"=w515, "stream index"=w512, "refnum in"=w516) -> ("error out"=w514:errorcluster, "refnum out"=w513:refnum<k20>)  [unwired: 7 in]
    n110 = Multiply(x="Record Size", y=u16 4) -> (x*y=w518:u16)
    n111 = call-poly <instrlib>:"Start Stream.vi"("error in (no error)"=w514, "num samples"=w518, "stream index"=w512, "refnum in"=w513) -> ("error out"=w532:errorcluster, "refnum out"=w530:refnum<k20>)  [unwired: 6 in]
    n112 = call-poly <instrlib>:"Wait.vi"("error in (no error)"=w532, "stream index"=w512, "refnum in"=w530) -> ("error out"=w528:errorcluster, "samples transferred"=w531:u64, "refnum out"=w529:refnum<k20>)  [unwired: 5 in, 1 out]
    n113 = xnode "Invoke Method"("FPGA VI Reference In"=w529, "error in"=w528, "Number of Elements"=w531) -> ("FPGA VI Reference Out"=w541:refnum<k20>, "error out"=w527:errorcluster, "Data"=w535:void[])  [unwired: 1 in, 1 out]
    n114 = call "Scale Acquired Data NI 5783.vi"("range (V)"=w521, "Sample Rate"=w522, "Number of Bits"=i16 16, "Data In"=w535) -> ("Data"=→"AI":waveform(dbl)[])  [unwired: 7 in]
    n115 = Or(x=w527) -> (x .or. y?=w538:bool)  [unwired: 1 in]
    n116 = in-place {
      in-place-border: [w544] -> w510
      in-place-border: w538 -> [w546]
      n117 = in-place-dvr #2(w539) -> (w545:bool, w543:errorcluster)
      n118 = Compound Arithmetic op=OR(w546, w545, w543) -> (w544:bool)
      n119 = in-place-dvr #2(w544) -> ()  [unwired: 2 out]
    }
    n120 = local read "stop"() -> (w509:bool)
    n121 = Or(x=w509, y=w510) -> (x .or. y?=w511:bool)
    n122 = Wait (ms)(milliseconds to wait=u32 100) -> ()  [unwired: 1 out]
  }
  n123 = Merge Errors(w1, w2) -> (w3:errorcluster)
  n124 = xnode "Read/Write Control"("FPGA VI Reference In"=w4, "error in"=w3, "stream.request state 2"=3) -> ("FPGA VI Reference Out"=w10:refnum<k20>, "error out"=w12:errorcluster)
  n125 = xnode "Close FPGA VI Reference"("FPGA VI Reference In"=w10, "error in"=w12) -> ("error out"=w19:errorcluster)
  n126 = call <vilib>:"Simple Error Handler.vi"("error in (no error)"=w19) -> ("error out"=→"Error Out":errorcluster)  [unwired: 4 in, 4 out]
